vi "Feedback Value.vi"(0 "Set Point":dbl, 1 "Invert Rotation":bool, 5 "Divisor":dbl=500.0 format="%#_13g", 7 "Addend":dbl=0.15 format="%#_13g", 9 "Deadband":dbl, 11 "Maximum Amplitude":dbl=0.5 format="%#_13g", 12 "Current Value":dbl) -> (8 "Rotation":dbl)   [LabVIEW 2015]
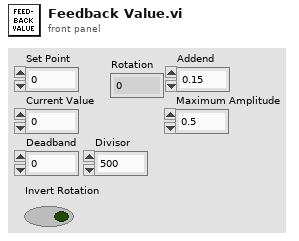
[diagram p1: front panel]
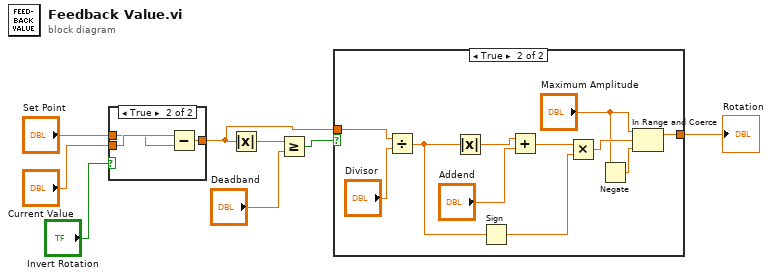
[diagram p0: block diagram]
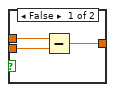
[diagram p2: hidden frame]
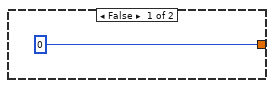
[diagram p3: hidden frame]
diagram:
  n1 = case shown="True" "Invert Rotation" {
    tunnel: [w11 w13] -> w8
    tunnel: "Current Value" -> [w10 w14]
    tunnel: "Set Point" -> [w9 w12]
    frame False {
      n2 = Subtract(x=w9, y=w10) -> (x-y=w11:dbl)
    }
    frame True {
      n3 = Subtract(x=w14, y=w12) -> (x-y=w13:dbl)
    }
  }
  n4 = Absolute Value(x=w8) -> (abs(x)=w6:dbl)
  n5 = Greater Or Equal?(x=w6, y="Deadband") -> (x >= y?=w7:bool)
  n6 = case shown="True" w7 {
    tunnel: [0 w26] -> w5
    tunnel: w8 -> [_ w24]
    frame False {
    }
    frame True {
      n7 = Divide(x=w24, y="Divisor") -> (x/y=w21:dbl)
      n8 = Absolute Value(x=w21) -> (abs(x)=w23:dbl)
      n9 = Sign(1:w21) -> (0:w20:dbl)
      n10 = Add(x=w23, y="Addend") -> (x+y=w19:dbl)
      n11 = Multiply(x=w19, y=w20) -> (x*y=w18:dbl)
      n12 = Negate(x="Maximum Amplitude") -> (-x=w17:dbl)
      n13 = In Range and Coerce(upper limit="Maximum Amplitude", x=w18, lower limit=w17) -> (coerced(x)=w26:dbl)  [unwired: 1 out]
    }
  }
  "Rotation" <- w5
